vi "Signature_Format_Save n Print Word Report (SubVI).vi"(5 "עבר/נכשל":string="עבר/נכשל", 7 "מפעיל":string="ANS", 8 "error in (no error)":errorcluster, 10 "Path":path, 11 "NI_report in":refnum<class "NI_report.lvclass">) -> ()   [LabVIEW 2015]
uses:
  <vilib>/Utility/NIReport.llb/NI_report.lvclass
  <vilib>/Utility/NIReport.llb/Append Report Text (str wrap).vi
  <vilib>/Utility/NIReport.llb/Word/NI_Word.lvclass
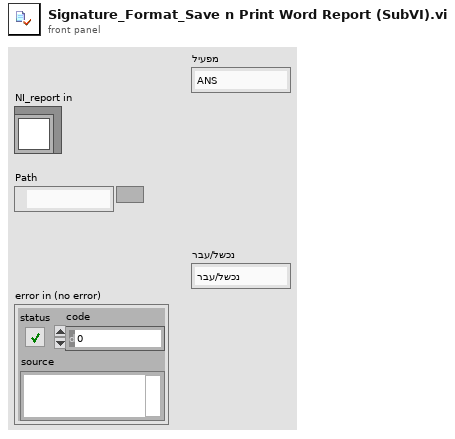
[diagram p1: front panel]
types:
  T1 = cluster{"alignment":enum16{"Left", "Centered", "Right", "Justify"}, "left":dbl, "right":dbl, "special":enum16{"(none)", "First line", "Hanging"}, "by":dbl, "before":dbl, "after":dbl, "line spacing":enum16{"Single", "1,5 lines", "Double", "At least", "Exactly", "Multiple"}, "at":dbl}
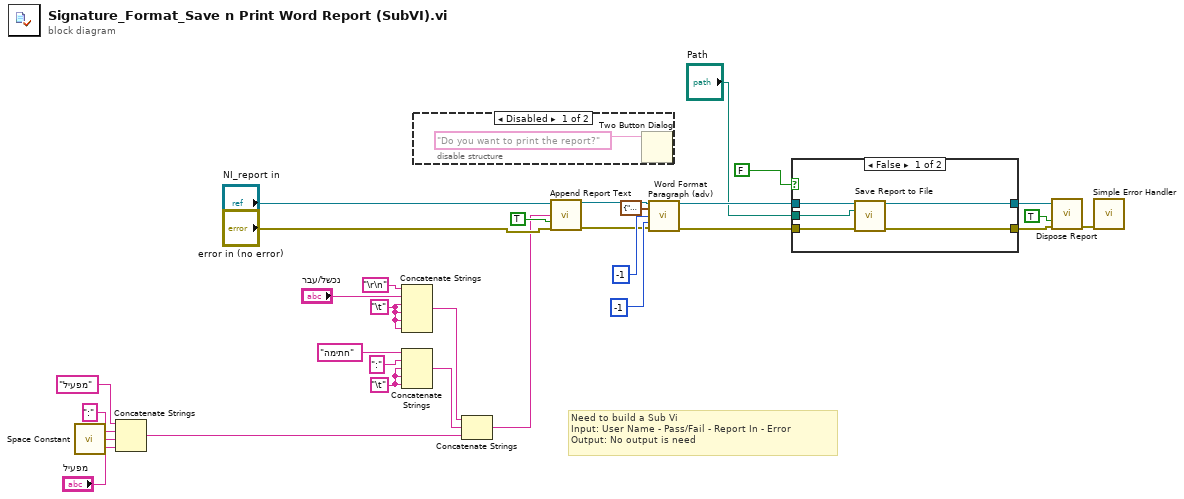
[diagram p0: block diagram]
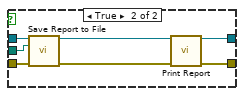
[diagram p3: hidden frame]
diagram:
  w13 = "\t"
  w2 = "\t"
  # "Need to build a Sub Vi\nInput: User Name - Pass/Fail - Report In - Error\nOutput: No output is need"
  n1 = call <vilib>:"Space Constant.vi"() -> ("String"=w4:string)
  n2 = Concatenate Strings("מפעיל" ("string"), ":" ("string"), w4, "מפעיל") -> (w10:string)
  n3 = Concatenate Strings("\r\n", "עבר/נכשל", w13, w13, w13, w13) -> (w12:string)
  n4 = Concatenate Strings("חתימה" ("string"), ":" ("string"), w2, w2, w2) -> (w9:string)
  n5 = disable-structure shown="Disabled" {
    frame Disabled {
      n6 = Two Button Dialog(message="Do you want to print the report?") -> ()  [unwired: 2 in, 1 out]
    }
    frame Enabled {
    }
  }
  n7 = Concatenate Strings(w12, w9, w10) -> (w1:string)
  n8 = call-poly <vilib>:"Append Report Text.vi"("report in"="NI_report in", "text"=w1, "append on new line? (F)"=TRUE, "error in (no error)"="error in (no error)") -> ("report out"=w25:refnum<class "NI_report.lvclass">, "error out"=w24:errorcluster)  [unwired: 8 in, 2 out]
  n9 = call <vilib>:"Word Format Paragraph (adv).vi"("report in"=w25, "indent and spacing"=T1 {"alignment"=enum."Centered", "left"=0.0, "right"=0.0, "special"=enum."(none)", "by"=0.0, "before"=0.0, "after"=0.0, "line spacing"=enum."Single", "at"=0.0}, "start (-1)"=-1, "end (-1)"=-1, "error in (no error)"=w24) -> ("report out"=w20:refnum<class "NI_report.lvclass">, "error out"=w19:errorcluster)  [unwired: 9 in]
  n10 = case shown="False" FALSE {
    tunnel: [w36 w42] -> w22
    tunnel: "Path" -> [w35 w43]
    tunnel: [w34 w40] -> w17
    tunnel: w20 -> [w33 w38]
    tunnel: w19 -> [w32 w37]
    frame False {
      n11 = call-dynamic "Save Report to File.vi"("report in"=w33, "report file path"=w35, "error in (no error)"=w32) -> ("report out"=w34:refnum<class "NI_report.lvclass">, "error out"=w36:errorcluster)  [unwired: 11 in]
    }
    frame True {
      n12 = call-dynamic "Save Report to File.vi"("report in"=w38, "report file path"=w43, "error in (no error)"=w37) -> ("report out"=w41:refnum<class "NI_report.lvclass">, "error out"=w39:errorcluster)  [unwired: 11 in]
      n13 = call-dynamic "Print Report.vi"("report in"=w41, "error in (no error)"=w39) -> ("report out"=w40:refnum<class "NI_report.lvclass">, "error out"=w42:errorcluster)  [unwired: 12 in]
    }
  }
  n14 = call-dynamic "Dispose Report.vi"("report in"=w17, "save changes? (F)"=TRUE, "error in (no error)"=w22) -> ("error out"=w23:errorcluster)  [unwired: 12 in]
  n15 = call <vilib>:"Simple Error Handler.vi"("error in (no error)"=w23) -> ()  [unwired: 4 in, 5 out]
